vi "LSX Set Zw Travel.vi"(8 "error in (no error)":errorcluster, 9 "dDistance":dbl, 10 "lIndex":i32, 11 "lLSID":i32) -> (0 "error out":errorcluster, 3 "function return":i32)   [LabVIEW 2018, in "Tango.lvlib"]
doc: "TANGOAPI int TANGOCALL LSX_SetZwTravel (int lLSID, int lIndex, double dDistance);"
uses:
  <userlib>/Tango/Tango.lvlib
  <userlib>/Tango/Tango_DLL.dll
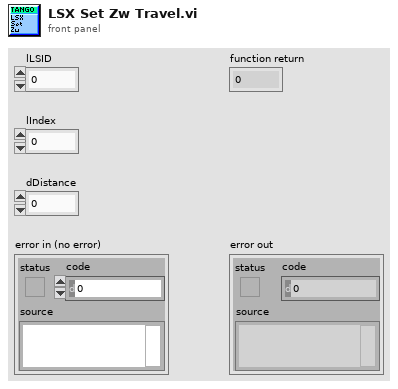
[diagram p1: front panel]
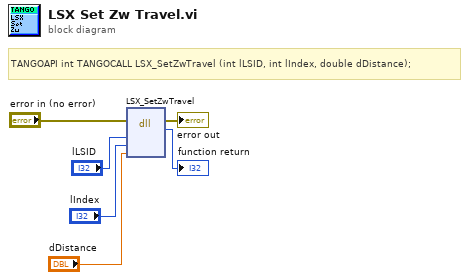
[diagram p0: block diagram]
diagram:
  # "TANGOAPI int TANGOCALL LSX_SetZwTravel (int lLSID, int lIndex, double dDistance);"
  n1 = dll-call lib="C:/Program Files (x86)/National Instruments/LabVIEW 2018/user.lib/Tango/Tango_DLL.*" fn="LSX_SetZwTravel"(error in="error in (no error)", "lLSID"="lLSID", "lIndex"="lIndex", "dDistance"="dDistance") -> (error out=→"error out":errorcluster, →"function return":i32)  [unwired: 5 in, 1 out]
